vi "art联动采集V4.5.vi"() -> ()   [LabVIEW 2016]
uses:
  <vilib>/Instr/_visa.llb/VISA Configure Serial Port (Instr).vi
  <vilib>/Utility/file.llb/Write Delimited Spreadsheet (DBL).vi
panel:
  in  "hDevice 2":i32
  in  "逐行扫描":bool
  in  "定位模式":bool
  in  "X终点":dbl
  in  "Y终点":dbl
  in  "高级设置":bool
  in  "Y轴回零速度":dbl=15000.0
  in  "X轴回零速度":dbl=15000.0
  in  "细分设置":dbl=8.0
  in  "等待时间":u32=40
  in  "文件保存":path=path "C:/Users/H301/Desktop/art采集实验数据" caption="保存路径"
  out "行用时（s）":dbl
  out "time（行）":u32
  out "error out":errorcluster caption="错误输出"
  in  "退出扫描(Esc)":bool
  in  "N_Length":i32=16384
  out "M_Length":i32
  out "hDevice":i32=241832032
  out "pulDDR2Length":u32=256
  out "总用时（s）":dbl
  out "毫秒计时值":u32=3586537
  out "数组":dbl[][](array[numeric])=[[58819.77200735986, 88200.32943600747]]
  out "强度图":dbl[][](graph)=[[58819.77200735986, 88200.32943600747]]
  out "judge":dbl
  out "Xloop":dbl
  out "幅频谱":dbl[](graph)
  out "时域谱":dbl[](graph)
  out "错误输出":errorcluster
  in  "启动":bool
  in  "逐点扫描":bool
  in  "X归零":bool
  in  "Y归零":bool
  in  "Y起点":dbl
  in  "Y轴速度":dbl=9000.0
  in  "X轴速度":dbl=9000.0
  out "电机状态":bool
  in  "电机端口":refnum<visa-resource-name>="COM6"
  out "Yloop":dbl=1.0
  out "X扫描范围":dbl=150.0
  out "Y扫描范围":dbl=75.0
  out "Y序":i32
  in  "X起点":dbl
  out "Y(mm)":dbl
  out "x+y 2":dbl=3.0
  in  "Y:":dbl=1.0
  in  "精度":dbl=0.001
  in  "电机急停":bool
  out "X（mm）":dbl
  out "x+y":dbl=1.0
  in  "X:":dbl=1.0
  # "实时坐标"
  # "时域谱"
  # "频域谱"
  # "归零"
  # "扫描区域"
  # "扫描步进(mm)"
  # "X:"
  # "~"
  # "Y:"
  # "~"
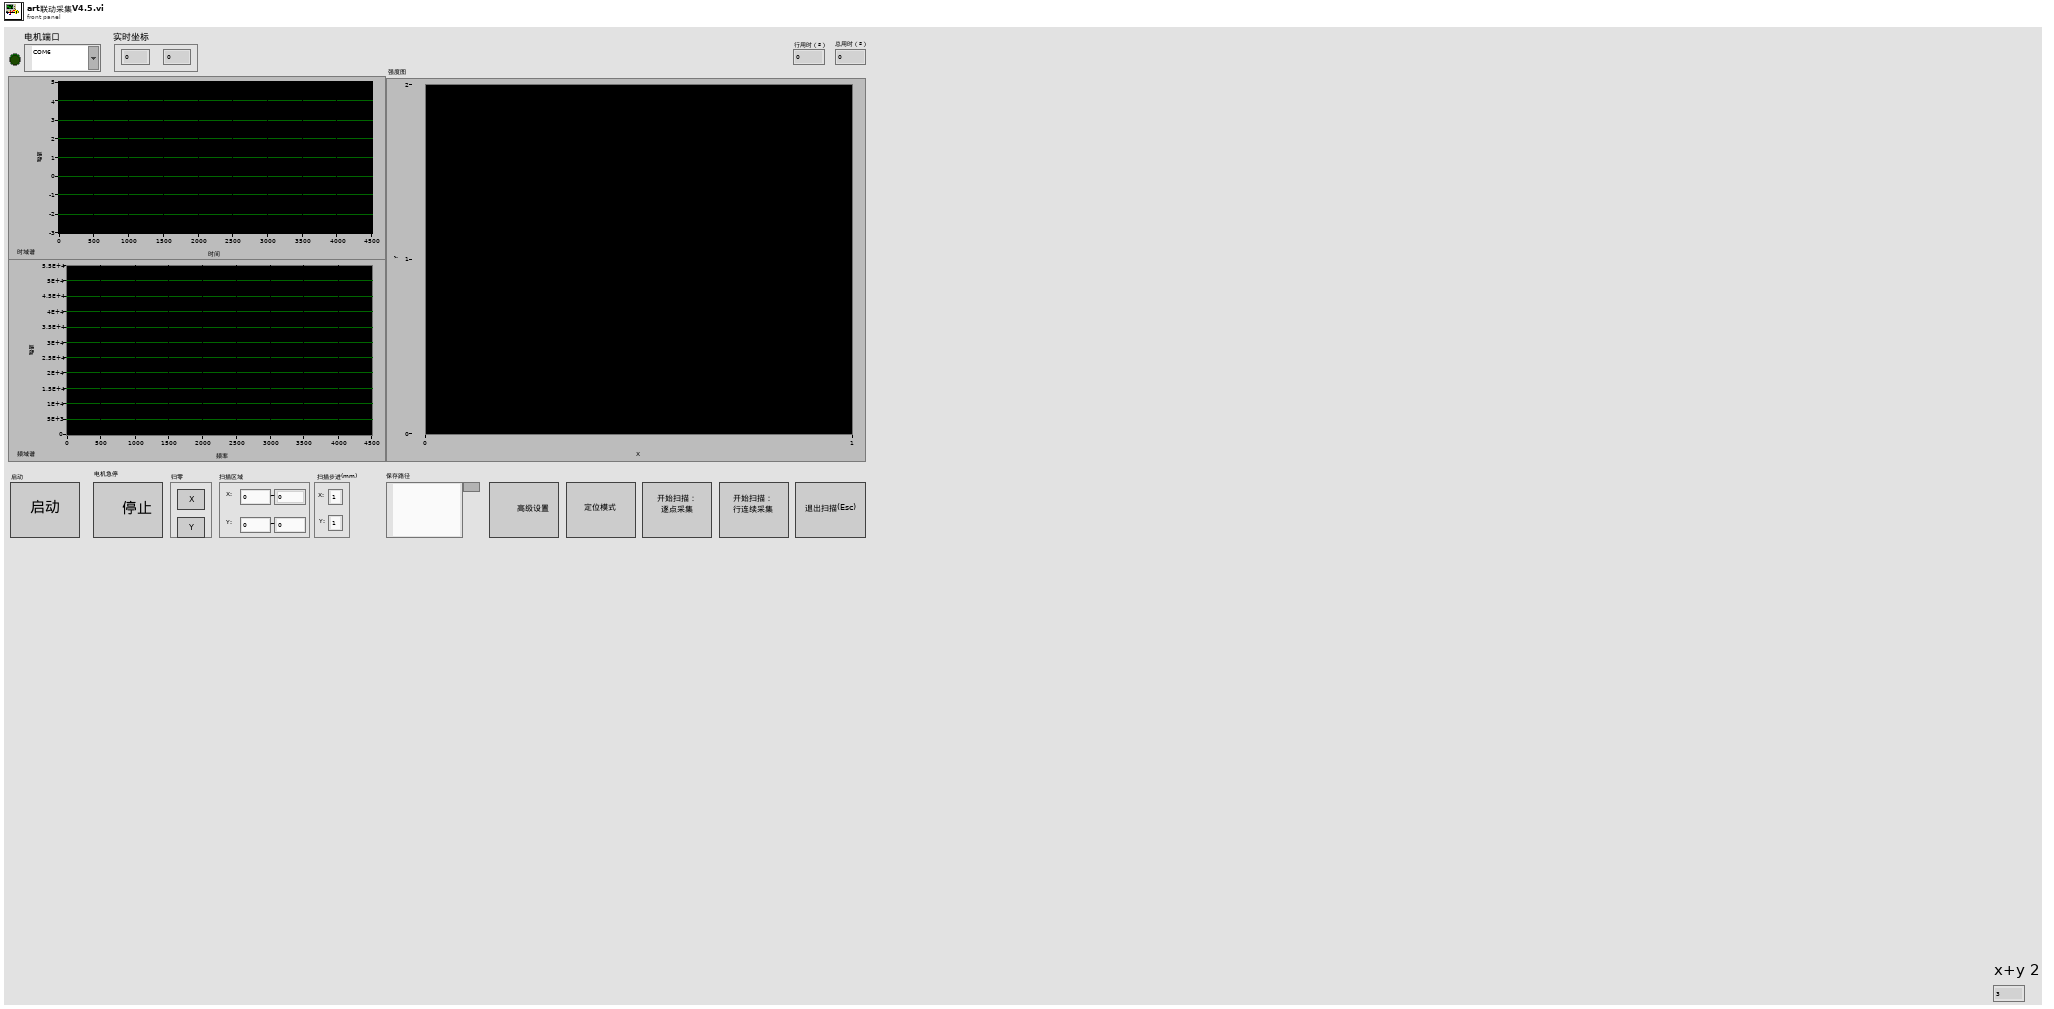
[diagram p1: front panel]
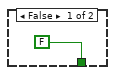
[diagram p2: hidden frame]
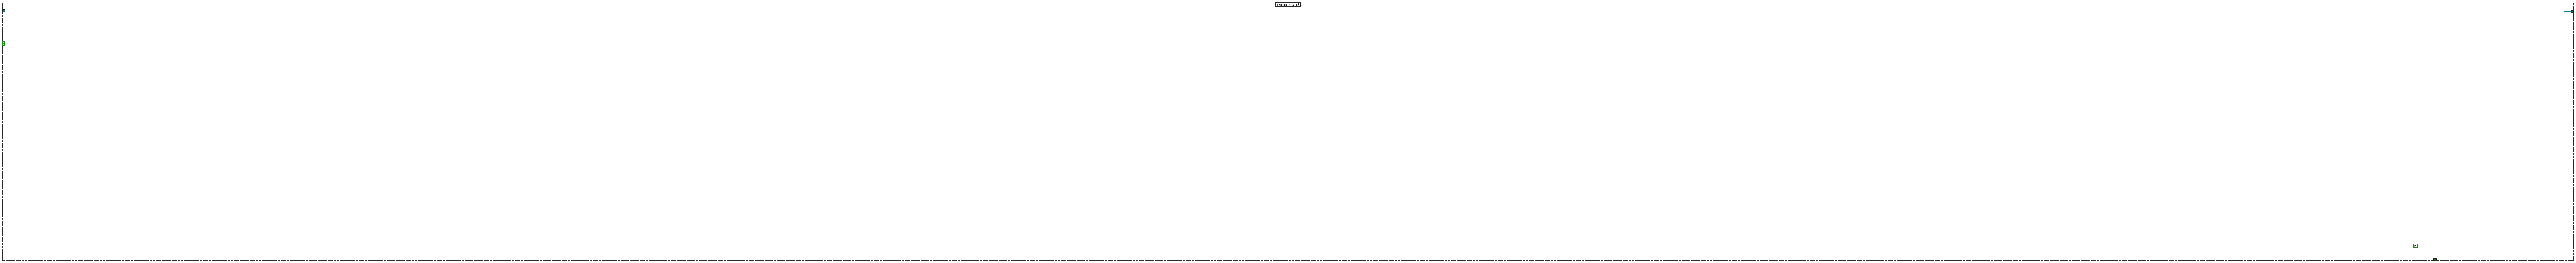
[diagram p3: hidden frame]
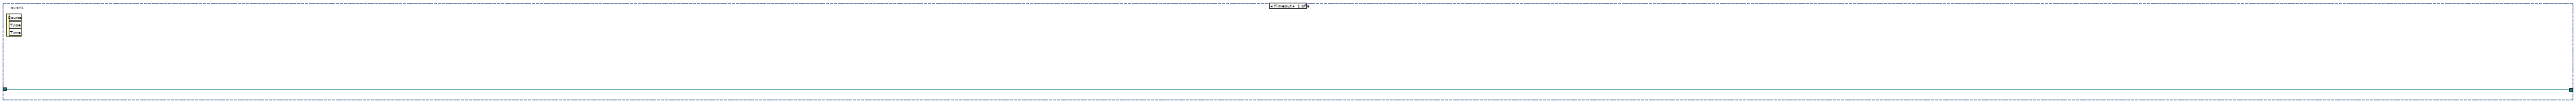
[diagram p4: hidden frame]
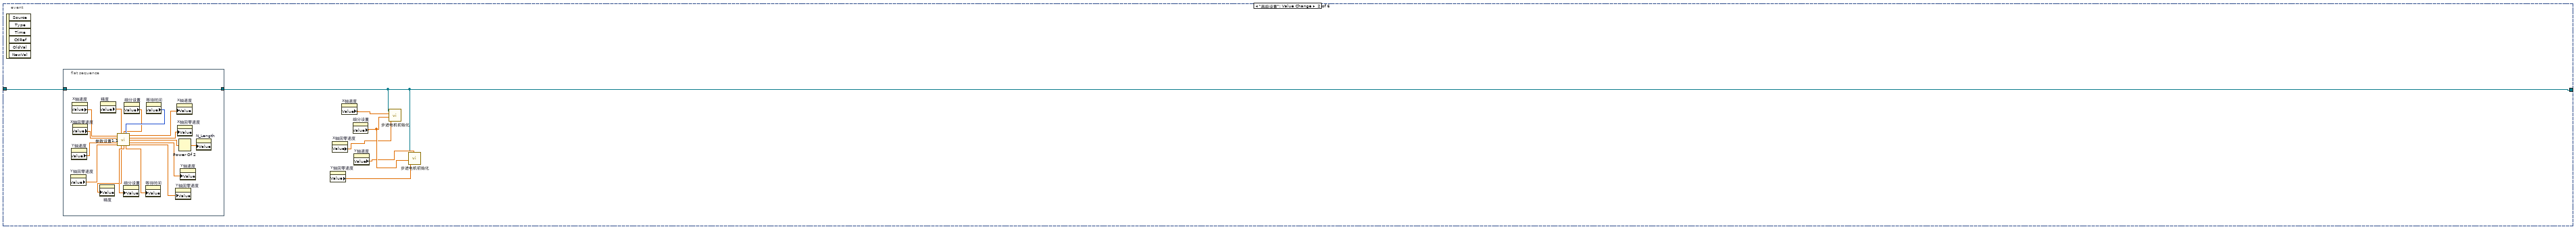
[diagram p5: hidden frame]
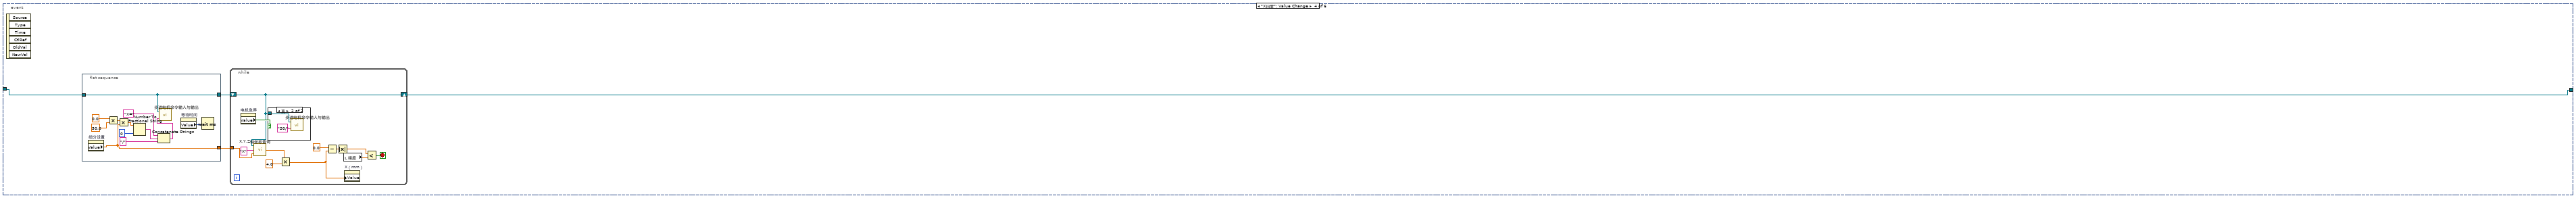
[diagram p6: hidden frame]
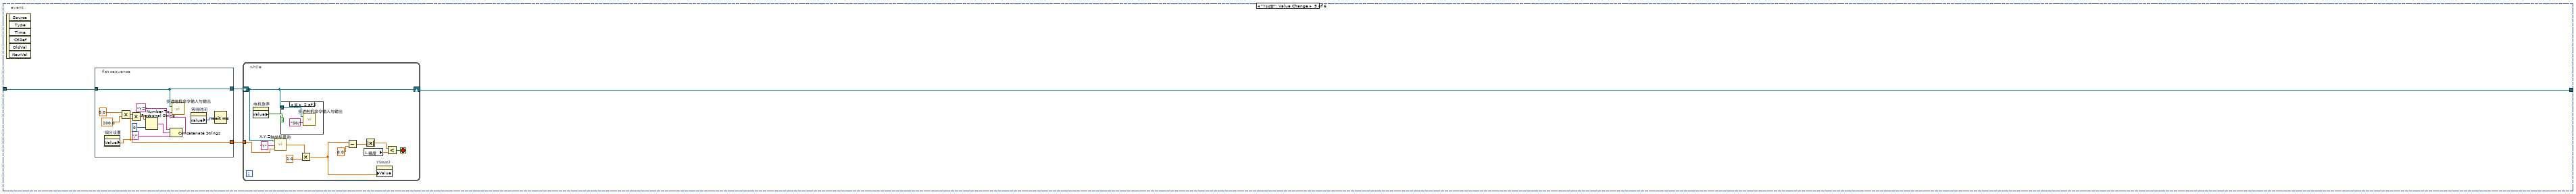
[diagram p8: hidden frame]
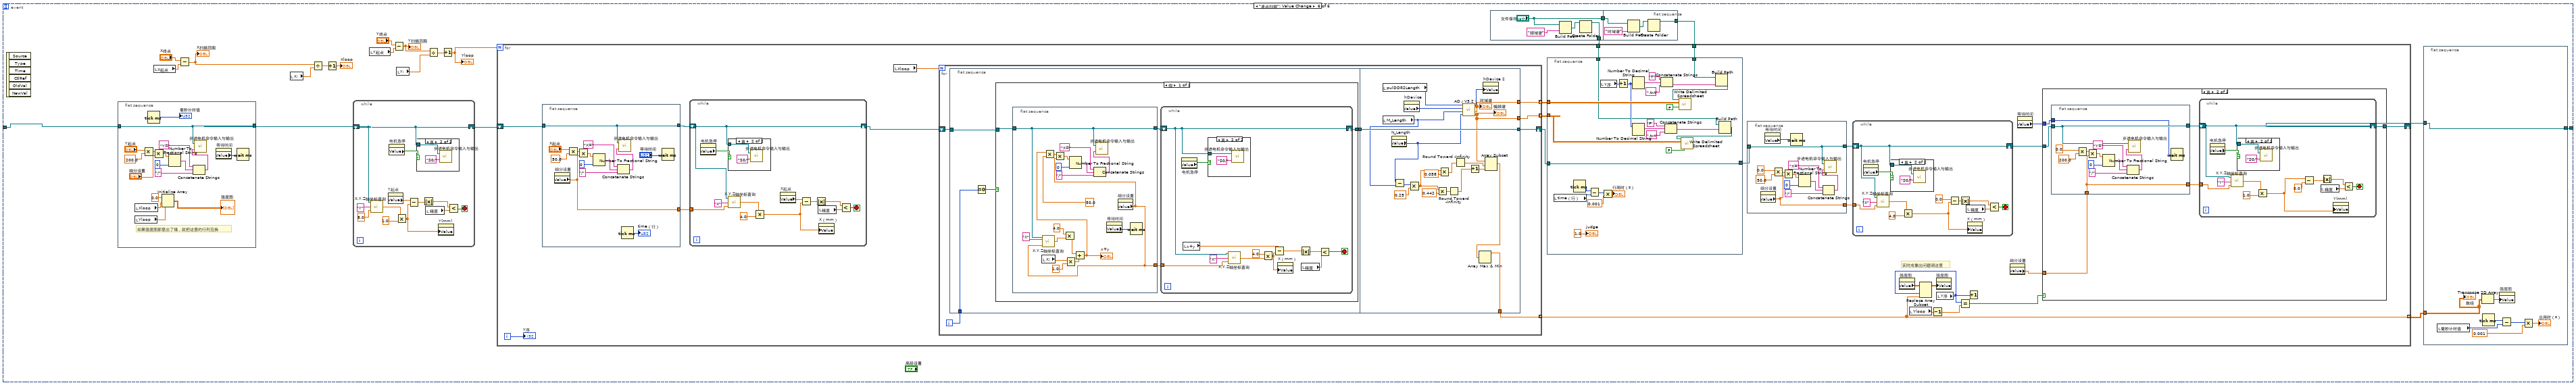
[diagram p10: hidden frame]
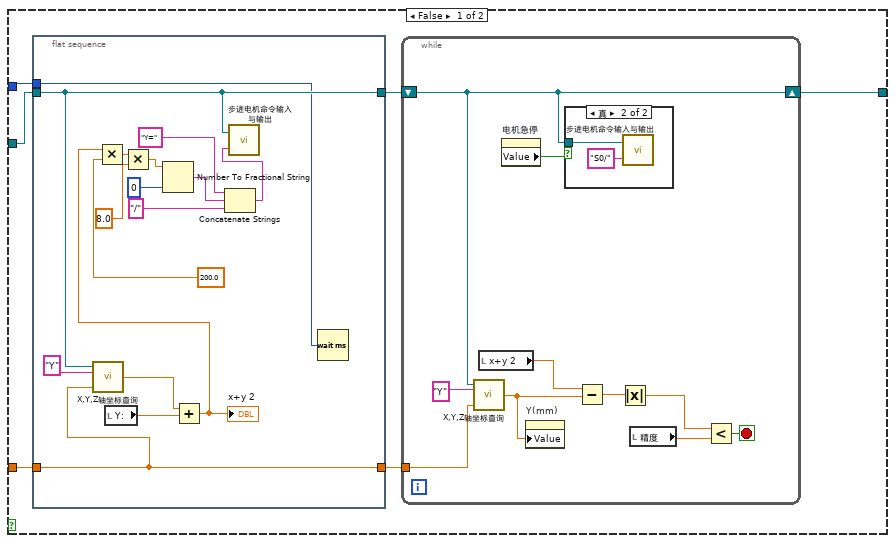
[diagram p14: hidden frame]
diagram:
  n1 = while {
    stop <- w3 stop-if-true
    n2 = case shown="真" "启动" {
      tunnel: [FALSE ("ESC") w12] -> w3
      frame False {
      }
      frame True {
        w25 = 0  # OutClockSource
        w26 = 0  # bClockSourceDir
        w28 = 10000000  # Frequency
        w29 = 0  # ClockSource
        w30 = 0  # TrigLevelVolt
        w18 = 1
        w31 = 0  # TriggerDir
        w32 = 0  # TriggerSource
        w33 = 0  # ATRTriggerChannel
        w34 = 0  # TriggerMode
        w19 = 0  # M_Length
        w35 = 1  # CouplingType
        w36 = 0  # DeviceLgcID
        w46 = u16 0 items=["无", "XON/XOFF", "RTS/CTS", "XON/XOFF & RTS/CTS", "DTR/DSR", "XON/XOFF & DTR/DSR"] ("flow control (0:none)")
        w47 = u16 10 items=["1.0"=10, "1.5"=15, "2.0"=20] ("stop bits (10: 1 bit)")
        # "3"
        # "2"
        # "1"
        n3 = call-poly "VISA Configure Serial Port"("VISA resource name"="电机端口", "baud rate (9600)"=u32 9600, "data bits (8)"=u16 8, "parity (0:none)"=enum16{"None", "Odd", "Even", "Mark", "Space"}."None", "stop bits (10: 1 bit)"=w47, "flow control (0:none)"=w46) -> ("VISA resource name out"=w38:refnum<visa-resource-name>, "error out"=→"error out":errorcluster)  [unwired: 1 in, 7 out]
        n4 = Build Array "InputRange"(w18, w18, w18, w18) -> (w17:i32[])
        n5 = dll-call lib="PTH2aabs CUsersH301Desktopart闭环扫描程序采集卡控制INFamd64PCI8502_32.dll" fn="PCI8502_CreateDevice" label="CreateDevice"("DeviceLgcID"=w36) -> (w23:i32)  [unwired: 4 in, 2 out]
        n6 = property on="细分设置" class="DigNum (严格)"() -> ("Value"=w11:dbl)  [unwired: 2 in, 2 out]
        n7 = Build Array (concatenate) "InitDeviceAD"(w28, w17, w35, w19, "N_Length", w34, w33, w32, w31, w30, w29, w26, w25) -> (w27:i32[])
        n8 = call "步进电机初始化.vi"("回零速度"="X轴回零速度", "细分设置"=w11, "X轴速度"="X轴速度", "串口通信端口"=w38) -> ()  [unwired: 2 in, 1 out]
        n9 = dll-call lib="PTH2aabs CUsersH301Desktopart闭环扫描程序采集卡控制INFamd64PCI8502_32.dll" fn="PCI8502_GetDDR2Length" label="GetDDR2Length"("hDevice"=w23, "pulDDR2Length"=u32 0) -> ("hDevice"=w22:i32, "pulDDR2Length"=→"pulDDR2Length":u32)  [unwired: 4 in, 2 out]
        n10 = call "步进电机初始化.vi"("Y轴速度"="Y轴速度", "回零速度"="Y轴回零速度", "细分设置"=w11, "串口通信端口"=w38) -> ()  [unwired: 2 in, 1 out]
        n11 = call "步进电机命令输入与输出.vi"("输入字符串"="?R/", "串口通信端口"=w38) -> ("返回字符串"=w43:string)
        n12 = dll-call lib="PTH2aabs CUsersH301Desktopart闭环扫描程序采集卡控制INFamd64PCI8502_32.dll" fn="PCI8502_InitDeviceAD" label="InitDeviceAD"("hDevice"=w22, "pADPara"=w27) -> ("hDevice"=→"hDevice":i32)  [unwired: 5 in, 2 out]
        n13 = String Subset(string=w43, offset (0)=0 ("偏移量(0)"), length (rest)=2 ("长度（剩余）")) -> (substring=w40:string)
        n14 = Equal?(x=w40, y="OK") -> (x = y?=w37:bool)
        "电机状态" <- w37
        n15 = case shown="真" w37 {
          tunnel: w38 -> [w53 w56]
          tunnel: [w53 w54] -> w13
          tunnel: [FALSE ("ESC") w55] -> w12
          frame False {
          }
          frame True {
            n16 = while {
              tunnel: ["退出扫描(Esc)"] -> w55
              shift-right: [w57] -> w54
              shift-left: w56 -> [w62]
              stop <- "退出扫描(Esc)" stop-if-true
              n17 = property on="高级设置" class="Bool"("Visible"=TRUE ("可见")) -> ()  [unwired: 2 in, 2 out]
              n18 = property on="定位模式" class="Bool"("Visible"=TRUE ("可见")) -> ()  [unwired: 2 in, 2 out]
              n19 = event shown="[2] \"定位模式\": 值改变" {
                selector: _ -> [_ _ _ _ _ _]
                dyn-events: _ -> [_ _ _ _ _ _]
                timeout: 1 -> [_ _ _ _ _ _]
                tunnel: w62 -> [w63 w70 w96 w100 w130 w177]
                tunnel: [w63 w64 w95 w98 w128 w171] -> w57
                event Timeout {
                  n20 = event-data() -> ()  [unwired: 1 in, 3 out]
                }
                event "高级设置": Value Change {
                  n21 = event-data() -> ()  [unwired: 1 in, 6 out]
                  n22 = flat-sequence {
                    tunnel: w70 -> [w73]
                    tunnel: [w73] -> w64
                    frame #0 {
                      n23 = property on="Y轴回零速度" class="DigNum (严格)"() -> ("Value"=w77:dbl)  [unwired: 2 in, 2 out]
                      n24 = property on="Y轴速度" class="DigNum (严格)"() -> ("Value"=w76:dbl)  [unwired: 2 in, 2 out]
                      n25 = property on="X轴速度" class="DigNum (严格)"() -> ("Value"=w74:dbl)  [unwired: 2 in, 2 out]
                      n26 = property on="X轴回零速度" class="DigNum (严格)"() -> ("Value"=w75:dbl)  [unwired: 2 in, 2 out]
                      n27 = property on="精度" class="DigNum (严格)"() -> ("Value"=w81:dbl)  [unwired: 2 in, 2 out]
                      n28 = property on="细分设置" class="DigNum (严格)"() -> ("Value"=w82:dbl)  [unwired: 2 in, 2 out]
                      n29 = property on="等待时间" class="DigNum (严格)"() -> ("Value"=w83:u32)  [unwired: 2 in, 2 out]
                      n30 = call "参数设置1.1.vi"("X轴速度"=w74, "精度"=w81, "细分设置"=w82, "等待时间"=w83, "X轴回零速度"=w75, "Y轴速度"=w76, "Y轴回零速度"=w77) -> ("X轴速度"=w84:dbl, "X轴回零速度"=w85:dbl, "采样阶"=w71:dbl, "Y轴速度"=w86:dbl, "精度"=w78:dbl, "细分设置"=w79:dbl, "等待时间"=w80:dbl, "Y轴回零速度"=w87:dbl)  [unwired: 1 in]
                      n31 = property on="精度" class="DigNum (严格)"("Value"=w78) -> ()  [unwired: 2 in, 2 out]
                      n32 = property on="细分设置" class="DigNum (严格)"("Value"=w79) -> ()  [unwired: 2 in, 2 out]
                      n33 = property on="等待时间" class="DigNum (严格)"("Value"=w80) -> ()  [unwired: 2 in, 2 out]
                      n34 = property on="Y轴回零速度" class="DigNum (严格)"("Value"=w87) -> ()  [unwired: 2 in, 2 out]
                      n35 = property on="X轴速度" class="DigNum (严格)"("Value"=w84) -> ()  [unwired: 2 in, 2 out]
                      n36 = property on="X轴回零速度" class="DigNum (严格)"("Value"=w85) -> ()  [unwired: 2 in, 2 out]
                      n37 = Power Of 2(x=w71) -> (2^x=w72:dbl)
                      n38 = property on="Y轴速度" class="DigNum (严格)"("Value"=w86) -> ()  [unwired: 2 in, 2 out]
                      n39 = property on="N_Length" class="DigNum (严格)"("Value"=w72) -> ()  [unwired: 2 in, 2 out]
                    }
                  }
                  n40 = property on="Y轴回零速度" class="DigNum (严格)"() -> ("Value"=w66:dbl)  [unwired: 2 in, 2 out]
                  n41 = property on="X轴回零速度" class="DigNum (严格)"() -> ("Value"=w67:dbl)  [unwired: 2 in, 2 out]
                  n42 = property on="X轴速度" class="DigNum (严格)"() -> ("Value"=w68:dbl)  [unwired: 2 in, 2 out]
                  n43 = property on="细分设置" class="DigNum (严格)"() -> ("Value"=w69:dbl)  [unwired: 2 in, 2 out]
                  n44 = property on="Y轴速度" class="DigNum (严格)"() -> ("Value"=w65:dbl)  [unwired: 2 in, 2 out]
                  n45 = call "步进电机初始化.vi"("回零速度"=w67, "细分设置"=w69, "X轴速度"=w68, "串口通信端口"=w64) -> ()  [unwired: 2 in, 1 out]
                  n46 = call "步进电机初始化.vi"("Y轴速度"=w65, "回零速度"=w66, "细分设置"=w69, "串口通信端口"=w64) -> ()  [unwired: 2 in, 1 out]
                }
                event "定位模式": Value Change {
                  n47 = event-data() -> ()  [unwired: 1 in, 6 out]
                  n48 = local read "pulDDR2Length"() -> (w92:u32)
                  n49 = local read "M_Length"() -> (w90:i32)
                  n50 = property on="hDevice" class="DigNum (严格)"() -> ("Value"=w91:i32)  [unwired: 2 in, 2 out]
                  n51 = property on="N_Length" class="DigNum (严格)"() -> ("Value"=w89:i32)  [unwired: 2 in, 2 out]
                  n52 = call "电机定位1.1.vi"("VISA I"=w96, "pulDDR2Length"=w92, "hDevice"=w91, "M-length"=w90, "N-length"=w89) -> ("hDevice out"=w88:i32, "VISA O"=w95:refnum<visa-resource-name>, "X"=w94:dbl, "Y"=w93:dbl)  [unwired: 11 in]
                  n53 = property on="hDevice 2" class="DigNum (严格)"("Value"=w88) -> ()  [unwired: 2 in, 2 out]
                  n54 = property on="X（mm）" class="DigNum (严格)"("Value"=w94) -> ()  [unwired: 2 in, 2 out]
                  n55 = property on="Y(mm)" class="DigNum (严格)"("Value"=w93) -> ()  [unwired: 2 in, 2 out]
                }
                event "X归零": Value Change {
                  n56 = event-data() -> ()  [unwired: 1 in, 6 out]
                  n57 = flat-sequence {
                    tunnel: w100 -> [w104]
                    tunnel: [w104] -> w99
                    tunnel: [w101] -> w97
                    frame #0 {
                      n58 = property on="细分设置" class="DigNum (严格)"() -> ("Value"=w101:dbl)  [unwired: 2 in, 2 out]
                      n59 = Multiply(x=0.0, y=50.0) -> (x*y=w107:dbl)
                      n60 = Multiply(x=w107, y=w101) -> (x*y=w112:dbl)
                      n61 = Number To Fractional String(number=w112, precision (6)=i16 0 ("精度(6)")) -> (F-format string=w110:string)  [unwired: 2 out]
                      n62 = Concatenate Strings("X=" ("字符串"), w110, "/" ("字符串")) -> (w105:string)
                      n63 = call "步进电机命令输入与输出.vi"("输入字符串"=w105, "串口通信端口"=w104) -> ()  [unwired: 1 out]
                      n64 = property on="等待时间" class="DigNum (严格)"() -> ("Value"=w102:u32)  [unwired: 2 in, 2 out]
                      n65 = Wait (ms)(milliseconds to wait=w102) -> ()  [unwired: 1 out]
                    }
                  }
                  n66 = while {
                    tunnel: w97 -> [w113]
                    shift-right: [w114] -> w98
                    shift-left: w99 -> [w114]
                    stop <- w120 stop-if-true
                    n67 = property on="电机急停" class="Bool (严格)"() -> ("Value"=w121:bool)  [unwired: 2 in, 2 out]
                    n68 = call "X,Y,Z轴坐标查询.vi"("细分设置"=w113, "查询坐标轴"="X", "串口通信端口"=w114) -> ("坐标(mm)"=w122:dbl)
                    n69 = case shown="真" w121 {
                      tunnel: w114 -> [_ w125]
                      frame False {
                      }
                      frame True {
                        n70 = call "步进电机命令输入与输出.vi"("输入字符串"="S0/", "串口通信端口"=w125) -> ()  [unwired: 1 out]
                      }
                    }
                    n71 = Multiply(x=w122, y=4.0 ("x")) -> (x*y=w118:dbl)
                    n72 = Subtract(x=0.0, y=w118) -> (x-y=w117:dbl)
                    n73 = Absolute Value(x=w117) -> (abs(x)=w116:dbl)
                    n74 = local read "精度"() -> (w119:dbl)
                    n75 = property on="X（mm）" class="DigNum (严格)"("Value"=w118) -> ()  [unwired: 2 in, 2 out]
                    n76 = Less?(x=w116, y=w119) -> (x < y?=w120:bool)
                  }
                }
                event "Y归零": Value Change {
                  n77 = event-data() -> ()  [unwired: 1 in, 6 out]
                  n78 = flat-sequence {
                    tunnel: w130 -> [w134]
                    tunnel: [w134] -> w129
                    tunnel: [w131] -> w127
                    frame #0 {
                      n79 = property on="细分设置" class="DigNum (严格)"() -> ("Value"=w131:dbl)  [unwired: 2 in, 2 out]
                      n80 = Multiply(x=0.0, y=200.0) -> (x*y=w137:dbl)
                      n81 = Multiply(x=w137, y=w131) -> (x*y=w142:dbl)
                      n82 = Number To Fractional String(number=w142, precision (6)=i16 0 ("精度(6)")) -> (F-format string=w140:string)  [unwired: 2 out]
                      n83 = Concatenate Strings("Y=" ("字符串"), w140, "/" ("字符串")) -> (w135:string)
                      n84 = call "步进电机命令输入与输出.vi"("输入字符串"=w135, "串口通信端口"=w134) -> ()  [unwired: 1 out]
                      n85 = property on="等待时间" class="DigNum (严格)"() -> ("Value"=w132:u32)  [unwired: 2 in, 2 out]
                      n86 = Wait (ms)(milliseconds to wait=w132) -> ()  [unwired: 1 out]
                    }
                  }
                  n87 = while {
                    tunnel: w127 -> [w143]
                    shift-right: [w144] -> w128
                    shift-left: w129 -> [w144]
                    stop <- w150 stop-if-true
                    n88 = property on="电机急停" class="Bool (严格)"() -> ("Value"=w151:bool)  [unwired: 2 in, 2 out]
                    n89 = call "X,Y,Z轴坐标查询.vi"("细分设置"=w143, "查询坐标轴"="Y", "串口通信端口"=w144) -> ("坐标(mm)"=w152:dbl)
                    n90 = case shown="真" w151 {
                      tunnel: w144 -> [_ w155]
                      frame False {
                      }
                      frame True {
                        n91 = call "步进电机命令输入与输出.vi"("输入字符串"="S0/", "串口通信端口"=w155) -> ()  [unwired: 1 out]
                      }
                    }
                    n92 = Multiply(x=w152, y=1.0 ("x")) -> (x*y=w148:dbl)
                    n93 = Subtract(x=w148, y=0.0 ("x")) -> (x-y=w146:dbl)
                    n94 = local read "精度"() -> (w149:dbl)
                    n95 = Absolute Value(x=w146) -> (abs(x)=w145:dbl)
                    n96 = property on="Y(mm)" class="DigNum (严格)"("Value"=w148) -> ()  [unwired: 2 in, 2 out]
                    n97 = Less?(x=w145, y=w149) -> (x < y?=w150:bool)
                  }
                }
                event "逐点扫描": Value Change {
                  n98 = event-data() -> ()  [unwired: 1 in, 6 out]
                  n99 = flat-sequence {
                    tunnel: w177 -> [w202]
                    tunnel: [w202] -> w167
                    frame #0 {
                      # "如果强度图那里出了错，就把这里的行列互换"
                      n100 = local read "Xloop"() -> (w197:dbl)
                      n101 = local read "Yloop"() -> (w196:dbl)
                      n102 = Multiply(x="Y起点", y=200.0) -> (x*y=w205:dbl)
                      n103 = Tick Count (ms)() -> (millisecond timer value=→"毫秒计时值":u32)
                      n104 = Multiply(x=w205, y="细分设置") -> (x*y=w210:dbl)
                      n105 = Initialize Array(0.0 ("元素"), w197, w196) -> (→"强度图":dbl[][])
                      n106 = Number To Fractional String(number=w210, precision (6)=i16 0 ("精度(6)")) -> (F-format string=w208:string)  [unwired: 2 out]
                      n107 = Concatenate Strings("Y=" ("字符串"), w208, "/" ("字符串")) -> (w203:string)
                      n108 = call "步进电机命令输入与输出.vi"("输入字符串"=w203, "串口通信端口"=w202) -> ()  [unwired: 1 out]
                      n109 = property on="等待时间" class="DigNum (严格)"() -> ("Value"=w194:u32)  [unwired: 2 in, 2 out]
                      n110 = Wait (ms)(milliseconds to wait=w194) -> ()  [unwired: 1 out]
                    }
                  }
                  n111 = local read "X起点"() -> (w163:dbl)
                  n112 = Subtract(x="X终点", y=w163) -> (x-y=w162:dbl)
                  "X扫描范围" <- w162
                  n113 = local read "X:"() -> (w170:dbl)
                  n114 = Divide(x=w162, y=w170) -> (x/y=w168:dbl)
                  n115 = Increment(x=w168) -> (x+1=→"Xloop":dbl)
                  n116 = while {
                    shift-right: [w211] -> w159
                    shift-left: w167 -> [w211]
                    stop <- w216 stop-if-true
                    n117 = call "X,Y,Z轴坐标查询.vi"("细分设置"=8.0, "查询坐标轴"="Y", "串口通信端口"=w211) -> ("坐标(mm)"=w218:dbl)
                    n118 = property on="Y起点" class="DigNum (严格)"() -> ("Value"=w220:dbl)  [unwired: 2 in, 2 out]
                    n119 = property on="电机急停" class="Bool (严格)"() -> ("Value"=w217:bool)  [unwired: 2 in, 2 out]
                    n120 = Multiply(x=w218, y=1.0 ("x")) -> (x*y=w214:dbl)
                    n121 = Subtract(x=w220, y=w214) -> (x-y=w213:dbl)
                    n122 = case shown="真" w217 {
                      tunnel: w211 -> [_ w223]
                      frame False {
                      }
                      frame True {
                        n123 = call "步进电机命令输入与输出.vi"("输入字符串"="S0/", "串口通信端口"=w223) -> ()  [unwired: 1 out]
                      }
                    }
                    n124 = Absolute Value(x=w213) -> (abs(x)=w212:dbl)
                    n125 = local read "精度"() -> (w215:dbl)
                    n126 = property on="Y(mm)" class="DigNum (严格)"("Value"=w214) -> ()  [unwired: 2 in, 2 out]
                    n127 = Less?(x=w212, y=w215) -> (x < y?=w216:bool)
                  }
                  n128 = local read "Y起点"() -> (w165:dbl)
                  n129 = Subtract(x="Y终点", y=w165) -> (x-y=w161:dbl)
                  "Y扫描范围" <- w161
                  n130 = local read "Y:"() -> (w176:dbl)
                  n131 = Divide(x=w161, y=w176) -> (x/y=w175:dbl)
                  n132 = Increment(x=w175) -> (x+1=w174:dbl)
                  "Yloop" <- w174
                  n133 = for {
                    N: w174 -> [_]
                    shift-right: [w247] -> w173
                    shift-left: w159 -> [w227]
                    tunnel: [w229] -> w172 mode=indexing
                    tunnel: w157 -> [w233]
                    tunnel: w160 -> [w232]
                    i -> [w248]
                    # "实时成像出问题调这里"
                    n134 = flat-sequence {
                      tunnel: w227 -> [w305]
                      tunnel: [w305] -> w246
                      tunnel: [w301] -> w237
                      frame #0 {
                        n135 = property on="细分设置" class="DigNum (严格)"() -> ("Value"=w301:dbl)  [unwired: 2 in, 2 out]
                        n136 = Multiply(x="X起点", y=50.0) -> (x*y=w308:dbl)
                        n137 = Multiply(x=w308, y=w301) -> (x*y=w313:dbl)
                        n138 = Number To Fractional String(number=w313, precision (6)=i16 0 ("精度(6)")) -> (F-format string=w311:string)  [unwired: 2 out]
                        n139 = Concatenate Strings("X=" ("字符串"), w311, "/" ("字符串")) -> (w306:string)
                        n140 = call "步进电机命令输入与输出.vi"("输入字符串"=w306, "串口通信端口"=w305) -> ()  [unwired: 1 out]
                        n141 = Tick Count (ms)() -> (millisecond timer value=→"time（行）":u32)
                        n142 = Wait (ms)(milliseconds to wait="等待时间") -> ()  [unwired: 1 out]
                      }
                    }
                    n143 = while {
                      tunnel: w237 -> [w315]
                      shift-right: [w314] -> w225
                      shift-left: w246 -> [w314]
                      stop <- w320 stop-if-true
                      n144 = property on="电机急停" class="Bool (严格)"() -> ("Value"=w321:bool)  [unwired: 2 in, 2 out]
                      n145 = case shown="真" w321 {
                        tunnel: w314 -> [_ w326]
                        frame False {
                        }
                        frame True {
                          n146 = call "步进电机命令输入与输出.vi"("输入字符串"="S0/", "串口通信端口"=w326) -> ()  [unwired: 1 out]
                        }
                      }
                      n147 = call "X,Y,Z轴坐标查询.vi"("细分设置"=w315, "查询坐标轴"="X", "串口通信端口"=w314) -> ("坐标(mm)"=w322:dbl)
                      n148 = Multiply(x=w322, y=4.0 ("x")) -> (x*y=w318:dbl)
                      n149 = property on="X起点" class="DigNum (严格)"() -> ("Value"=w324:dbl)  [unwired: 2 in, 2 out]
                      n150 = Subtract(x=w324, y=w318) -> (x-y=w317:dbl)
                      n151 = Absolute Value(x=w317) -> (abs(x)=w316:dbl)
                      n152 = local read "精度"() -> (w319:dbl)
                      n153 = property on="X（mm）" class="DigNum (严格)"("Value"=w318) -> ()  [unwired: 2 in, 2 out]
                      n154 = Less?(x=w316, y=w319) -> (x < y?=w320:bool)
                    }
                    n155 = local read "Xloop"() -> (w238:dbl)
                    n156 = for {
                      N: w238 -> [_]
                      shift-right: [w399] -> w226
                      shift-left: w225 -> [w394]
                      tunnel: [w398] -> w245 mode=indexing
                      tunnel: [w397] -> w244 mode=indexing
                      tunnel: [w396] -> w229 mode=indexing
                      i -> [w395]
                      n157 = flat-sequence {
                        tunnel: w394 -> [w404]
                        tunnel: [w403] -> w400
                        tunnel: w395 -> [w401]
                        tunnel: [w462] -> w399
                        tunnel: w400 -> [w462]
                        tunnel: [w461] -> w398
                        tunnel: [w460] -> w397
                        tunnel: [w458] -> w396
                        frame #0 {
                          n158 = Equal To 0?(x=w401) -> (x = 0?=w402:bool)
                          n159 = case shown="假" w402 {
                            tunnel: w404 -> [w407 w442]
                            tunnel: [w406 w442] -> w403
                            frame False {
                              n160 = flat-sequence {
                                tunnel: w407 -> [w417]
                                tunnel: [w417] -> w408
                                tunnel: [w409] -> w405
                                frame #0 {
                                n161 = local read "X:"() -> (w411:dbl)
                                n162 = Multiply(x=w411, y=1.0 ("x")) -> (x*y=w416:dbl)
                                n163 = property on="等待时间" class="DigNum (严格)"() -> ("Value"=w410:u32)  [unwired: 2 in, 2 out]
                                n164 = property on="细分设置" class="DigNum (严格)"() -> ("Value"=w409:dbl)  [unwired: 2 in, 2 out]
                                n165 = call "X,Y,Z轴坐标查询.vi"("细分设置"=w409, "查询坐标轴"="X", "串口通信端口"=w417) -> ("坐标(mm)"=w413:dbl)
                                n166 = Multiply(x=4.0, y=w413) -> (x*y=w412:dbl)
                                n167 = Add(x=w412, y=w416) -> (x+y=w419:dbl)
                                "x+y" <- w419
                                n168 = Multiply(x=w419, y=50.0) -> (x*y=w422:dbl)
                                n169 = Multiply(x=w422, y=w409) -> (x*y=w427:dbl)
                                n170 = Number To Fractional String(number=w427, precision (6)=i16 0 ("精度(6)")) -> (F-format string=w425:string)  [unwired: 2 out]
                                n171 = Concatenate Strings("X=" ("字符串"), w425, "/" ("字符串")) -> (w420:string)
                                n172 = call "步进电机命令输入与输出.vi"("输入字符串"=w420, "串口通信端口"=w417) -> ()  [unwired: 1 out]
                                n173 = Wait (ms)(milliseconds to wait=w410) -> ()  [unwired: 1 out]
                                }
                              }
                              n174 = while {
                                tunnel: w405 -> [w428]
                                shift-right: [w437] -> w406
                                shift-left: w408 -> [w437]
                                stop <- w436 stop-if-true
                                n175 = property on="电机急停" class="Bool (严格)"() -> ("Value"=w434:bool)  [unwired: 2 in, 2 out]
                                n176 = local read "x+y"() -> (w438:dbl)
                                n177 = case shown="真" w434 {
                                tunnel: w437 -> [_ w440]
                                frame False {
                                }
                                frame True {
                                n178 = call "步进电机命令输入与输出.vi"("输入字符串"="S0/", "串口通信端口"=w440) -> ()  [unwired: 1 out]
                                }
                                }
                                n179 = call "X,Y,Z轴坐标查询.vi"("细分设置"=w428, "查询坐标轴"="X", "串口通信端口"=w437) -> ("坐标(mm)"=w432:dbl)
                                n180 = Multiply(x=4.0, y=w432) -> (x*y=w431:dbl)
                                n181 = Subtract(x=w438, y=w431) -> (x-y=w430:dbl)
                                n182 = property on="X（mm）" class="DigNum (严格)"("Value"=w431) -> ()  [unwired: 2 in, 2 out]
                                n183 = Absolute Value(x=w430) -> (abs(x)=w429:dbl)
                                n184 = local read "精度"() -> (w433:dbl)
                                n185 = Less?(x=w429, y=w433) -> (x < y?=w436:bool)
                              }
                            }
                            frame True {
                            }
                          }
                        }
                        frame #1 {
                          n186 = local read "pulDDR2Length"() -> (w457:u32)
                          n187 = local read "M_Length"() -> (w456:i32)
                          n188 = property on="N_Length" class="DigNum (严格)"() -> ("Value"=w445:i32)  [unwired: 2 in, 2 out]
                          n189 = Subtract(x=w445, y=w456) -> (x-y=w454:i32)
                          n190 = property on="hDevice" class="DigNum (严格)"() -> ("Value"=w443:i32)  [unwired: 2 in, 2 out]
                          n191 = Multiply(x=w454, y=0.25) -> (x*y=w447:dbl)
                          n192 = Multiply(x=w447, y=0.442) -> (x*y=w449:dbl)
                          n193 = Multiply(x=w447, y=0.058) -> (x*y=w451:dbl)
                          n194 = Round Toward -Infinity(1:w449) -> (0:w446:dbl)
                          n195 = Round Toward -Infinity(1:w451) -> (0:w450:dbl)
                          n196 = call "AD（V3.2）.vi"("N-length"=w445, "M-length"=w456, "hDevice"=w443, "pulDDR2Length"=w457) -> ("幅频谱"=w460:dbl[], "时域谱"=w461:dbl[], "hDevice out"=w444:i32)  [unwired: 5 in]
                          "时域谱" <- w461
                          "幅频谱" <- w460
                          n197 = Increment(x=w446) -> (x+1=w453:dbl)
                          n198 = property on="hDevice 2" class="DigNum (严格)"("Value"=w444) -> ()  [unwired: 2 in, 2 out]
                          n199 = Array Subset(array=w460, index=w450, length=w453) -> (w459:dbl[])
                          n200 = Array Max & Min(array=w459) -> (max value=w458:dbl)  [unwired: 3 out]
                        }
                      }
                    }
                    n201 = flat-sequence {
                      tunnel: w244 -> [w282]
                      tunnel: w245 -> [w290]
                      tunnel: w226 -> [w299]
                      tunnel: [w299] -> w240
                      tunnel: w233 -> [w277]
                      tunnel: w232 -> [w276]
                      frame #0 {
                        n202 = local read "time（行）"() -> (w298:u32)
                        n203 = Tick Count (ms)() -> (millisecond timer value=w294:u32)
                        n204 = Subtract(x=w294, y=w298) -> (x-y=w297:u32)
                        n205 = local read "Y序"() -> (w278:i32)
                        n206 = Multiply(x=w297, y=0.001) -> (x*y=→"行用时（s）":dbl)
                        n207 = Increment(x=w278) -> (x+1=w279:i32)
                        n208 = Number To Decimal String(number=w279) -> (decimal integer string=w288:string)  [unwired: 1 in]
                        n209 = Number To Decimal String(number=w279) -> (decimal integer string=w287:string)  [unwired: 1 in]
                        n210 = Concatenate Strings("T" ("字符串"), w288, ".txt" ("字符串")) -> (w291:string)
                        n211 = Concatenate Strings("F" ("字符串"), w287, ".txt" ("字符串")) -> (w285:string)
                        n212 = Build Path(base path=w277, name or relative path=w291) -> (appended path=w293:path)
                        n213 = call-poly <vilib>:"Write Delimited Spreadsheet.vi"("file path (dialog if empty)"=w293, "2D data"=w290, "transpose? (no:F)"=FALSE) -> ()  [unwired: 11 in, 2 out]
                        n214 = Build Path(base path=w276, name or relative path=w285) -> (appended path=w283:path)
                        n215 = call-poly <vilib>:"Write Delimited Spreadsheet.vi"("file path (dialog if empty)"=w283, "2D data"=w282, "transpose? (no:F)"=FALSE) -> ()  [unwired: 11 in, 2 out]
                        "judge" <- 1.0
                      }
                    }
                    n216 = flat-sequence {
                      tunnel: w240 -> [w253]
                      tunnel: [w253] -> w241
                      tunnel: [w251] -> w236
                      frame #0 {
                        n217 = property on="细分设置" class="DigNum (严格)"() -> ("Value"=w251:dbl)  [unwired: 2 in, 2 out]
                        n218 = property on="等待时间" class="DigNum (严格)"() -> ("Value"=w250:u32)  [unwired: 2 in, 2 out]
                        n219 = Multiply(x=0.0, y=50.0) -> (x*y=w256:dbl)
                        n220 = Multiply(x=w256, y=w251) -> (x*y=w261:dbl)
                        n221 = Wait (ms)(milliseconds to wait=w250) -> ()  [unwired: 1 out]
                        n222 = Number To Fractional String(number=w261, precision (6)=i16 0 ("精度(6)")) -> (F-format string=w259:string)  [unwired: 2 out]
                        n223 = Concatenate Strings("X=" ("字符串"), w259, "/" ("字符串")) -> (w254:string)
                        n224 = call "步进电机命令输入与输出.vi"("输入字符串"=w254, "串口通信端口"=w253) -> ()  [unwired: 1 out]
                      }
                    }
                    n225 = while {
                      tunnel: w236 -> [w262]
                      shift-right: [w263] -> w239
                      shift-left: w241 -> [w263]
                      stop <- w269 stop-if-true
                      n226 = property on="电机急停" class="Bool (严格)"() -> ("Value"=w270:bool)  [unwired: 2 in, 2 out]
                      n227 = call "X,Y,Z轴坐标查询.vi"("细分设置"=w262, "查询坐标轴"="X", "串口通信端口"=w263) -> ("坐标(mm)"=w271:dbl)
                      n228 = case shown="真" w270 {
                        tunnel: w263 -> [_ w274]
                        frame False {
                        }
                        frame True {
                          n229 = call "步进电机命令输入与输出.vi"("输入字符串"="S0/", "串口通信端口"=w274) -> ()  [unwired: 1 out]
                        }
                      }
                      n230 = Multiply(x=w271, y=4.0 ("x")) -> (x*y=w267:dbl)
                      n231 = Subtract(x=0.0, y=w267) -> (x-y=w266:dbl)
                      n232 = Absolute Value(x=w266) -> (abs(x)=w265:dbl)
                      n233 = local read "精度"() -> (w268:dbl)
                      n234 = property on="X（mm）" class="DigNum (严格)"("Value"=w267) -> ()  [unwired: 2 in, 2 out]
                      n235 = Less?(x=w265, y=w268) -> (x < y?=w269:bool)
                    }
                    n236 = property on="强度图" class="IntGraph (严格)"() -> ("Value"=w230:dbl[][])  [unwired: 2 in, 2 out]
                    n237 = local read "Yloop"() -> (w242:dbl)
                    n238 = Decrement(x=w242) -> (x-1=w243:dbl)
                    n239 = local read "Y序"() -> (w228:i32)
                    n240 = Replace Array Subset(array=w230, new element=w229, index (col)=w228) -> (w231:dbl[][])  [unwired: 1 in]
                    n241 = property on="强度图" class="IntGraph (严格)"("Value"=w231) -> ()  [unwired: 2 in, 2 out]
                    n242 = Equal?(x=w228, y=w243) -> (x = y?=w249:bool)
                    n243 = Increment(x=w228) -> ()  [unwired: 1 out]
                    n244 = property on="细分设置" class="DigNum (严格)"() -> ("Value"=w234:dbl)  [unwired: 2 in, 2 out]
                    n245 = property on="等待时间" class="DigNum (严格)"() -> ("Value"=w235:u32)  [unwired: 2 in, 2 out]
                    n246 = case shown="真" w249 {
                      tunnel: w239 -> [w333 w365]
                      tunnel: [w331 w366] -> w247
                      tunnel: w235 -> [w329 w363]
                      tunnel: w234 -> [w328 w362]
                      frame False {
                        n247 = flat-sequence {
                          tunnel: w333 -> [w336]
                          tunnel: [w336] -> w332
                          tunnel: [w334] -> w330
                          tunnel: w329 -> [w335]
                          tunnel: w328 -> [w334]
                          frame #0 {
                            n248 = call "X,Y,Z轴坐标查询.vi"("细分设置"=w334, "查询坐标轴"="Y", "串口通信端口"=w336) -> ("坐标(mm)"=w338:dbl)
                            n249 = local read "Y:"() -> (w337:dbl)
                            n250 = Add(x=w338, y=w337) -> (x+y=w340:dbl)
                            "x+y 2" <- w340
                            n251 = Multiply(x=w340, y=200.0) -> (x*y=w344:dbl)
                            n252 = Multiply(x=w344, y=8.0 ("细分设置")) -> (x*y=w349:dbl)
                            n253 = Number To Fractional String(number=w349, precision (6)=i16 0 ("精度(6)")) -> (F-format string=w347:string)  [unwired: 2 out]
                            n254 = Concatenate Strings("Y=" ("字符串"), w347, "/" ("字符串")) -> (w342:string)
                            n255 = call "步进电机命令输入与输出.vi"("输入字符串"=w342, "串口通信端口"=w336) -> ()  [unwired: 1 out]
                            n256 = Wait (ms)(milliseconds to wait=w335) -> ()  [unwired: 1 out]
                          }
                        }
                        n257 = while {
                          tunnel: w330 -> [w350]
                          shift-right: [w351] -> w331
                          shift-left: w332 -> [w351]
                          stop <- w357 stop-if-true
                          n258 = call "X,Y,Z轴坐标查询.vi"("细分设置"=w350, "查询坐标轴"="Y", "串口通信端口"=w351) -> ("坐标(mm)"=w355:dbl)
                          n259 = local read "x+y 2"() -> (w358:dbl)
                          n260 = property on="电机急停" class="Bool (严格)"() -> ("Value"=w354:bool)  [unwired: 2 in, 2 out]
                          n261 = property on="Y(mm)" class="DigNum (严格)"("Value"=w355) -> ()  [unwired: 2 in, 2 out]
                          n262 = case shown="真" w354 {
                            tunnel: w351 -> [_ w360]
                            frame False {
                            }
                            frame True {
                              n263 = call "步进电机命令输入与输出.vi"("输入字符串"="S0/", "串口通信端口"=w360) -> ()  [unwired: 1 out]
                            }
                          }
                          n264 = Subtract(x=w358, y=w355) -> (x-y=w353:dbl)
                          n265 = Absolute Value(x=w353) -> (abs(x)=w352:dbl)
                          n266 = local read "精度"() -> (w356:dbl)
                          n267 = Less?(x=w352, y=w356) -> (x < y?=w357:bool)
                        }
                      }
                      frame True {
                        n268 = flat-sequence {
                          tunnel: [w370] -> _
                          tunnel: [w370] -> w367
                          tunnel: w365 -> [w370]
                          tunnel: [w368] -> w364
                          tunnel: w363 -> [w369]
                          tunnel: w362 -> [w368]
                          frame #0 {
                            n269 = Multiply(x=0.0, y=200.0) -> (x*y=w374:dbl)
                            n270 = Multiply(x=w374, y=w368) -> (x*y=w379:dbl)
                            n271 = Number To Fractional String(number=w379, precision (6)=i16 0 ("精度(6)")) -> (F-format string=w377:string)  [unwired: 2 out]
                            n272 = Concatenate Strings("Y=" ("字符串"), w377, "/" ("字符串")) -> (w372:string)
                            n273 = call "步进电机命令输入与输出.vi"("输入字符串"=w372, "串口通信端口"=w370) -> ()  [unwired: 1 out]
                            n274 = Wait (ms)(milliseconds to wait=w369) -> ()  [unwired: 1 out]
                          }
                        }
                        n275 = while {
                          tunnel: w364 -> [w380]
                          shift-right: [w381] -> w366
                          shift-left: w367 -> [w381]
                          stop <- w387 stop-if-true
                          n276 = property on="电机急停" class="Bool (严格)"() -> ("Value"=w388:bool)  [unwired: 2 in, 2 out]
                          n277 = call "X,Y,Z轴坐标查询.vi"("细分设置"=w380, "查询坐标轴"="Y", "串口通信端口"=w381) -> ("坐标(mm)"=w389:dbl)
                          n278 = case shown="真" w388 {
                            tunnel: w381 -> [_ w392]
                            frame False {
                            }
                            frame True {
                              n279 = call "步进电机命令输入与输出.vi"("输入字符串"="S0/", "串口通信端口"=w392) -> ()  [unwired: 1 out]
                            }
                          }
                          n280 = Multiply(x=w389, y=1.0 ("x")) -> (x*y=w385:dbl)
                          n281 = Subtract(x=w385, y=0.0 ("x")) -> (x-y=w383:dbl)
                          n282 = local read "精度"() -> (w386:dbl)
                          n283 = Absolute Value(x=w383) -> (abs(x)=w382:dbl)
                          n284 = property on="Y(mm)" class="DigNum (严格)"("Value"=w385) -> ()  [unwired: 2 in, 2 out]
                          n285 = Less?(x=w382, y=w386) -> (x < y?=w387:bool)
                        }
                      }
                    }
                    "Y序" <- w248
                  }
                  n286 = flat-sequence {
                    tunnel: [w178] -> w160
                    tunnel: ["文件保存"] -> w158
                    tunnel: w158 -> [w183]
                    tunnel: [w182] -> w157
                    frame #0 {
                      n287 = Build Path(base path="文件保存", name or relative path="频域谱" ("名称或相对路径")) -> (appended path=w181:path)
                      n288 = Create Folder(path (use dialog)=w181) -> (created path=w178:path)  [unwired: 2 in, 2 out]
                    }
                    frame #1 {
                      n289 = Build Path(base path=w183, name or relative path="时域谱" ("名称或相对路径")) -> (appended path=w184:path)
                      n290 = Create Folder(path (use dialog)=w184) -> (created path=w182:path)  [unwired: 2 in, 2 out]
                    }
                  }
                  n291 = flat-sequence {
                    tunnel: w173 -> [w188]
                    tunnel: w172 -> [w187]
                    tunnel: [w188] -> w171
                    frame #0 {
                      n292 = local read "毫秒计时值"() -> (w192:u32)
                      n293 = Transpose 2D Array(2D array=w187) -> (transposed array=w186:dbl[][])
                      n294 = Tick Count (ms)() -> (millisecond timer value=w193:u32)
                      n295 = property on="强度图" class="IntGraph (严格)"("Value"=w186) -> ()  [unwired: 2 in, 2 out]
                      n296 = Subtract(x=w193, y=w192) -> (x-y=w189:u32)
                      n297 = Multiply(x=w189, y=0.001) -> (x*y=→"总用时（s）":dbl)
                      "数组" <- w187
                    }
                  }
                }
              }
            }
          }
        }
        n298 = dll-call lib="PTH2]abs CUsersH301Desktopart闭环扫描程序采集卡控制INFamd64\nPCI8502_32" fn="PCI8502_ReleaseDeviceAD" label="ReleaseDeviceAD"("hDevice"="hDevice 2") -> ("hDevice"=w15:i32)  [unwired: 4 in, 2 out]
        n299 = VISA Close(VISA resource name=w13) -> (error out=→"错误输出":errorcluster)  [unwired: 1 in]
        n300 = dll-call lib="PTH2]abs CUsersH301Desktopart闭环扫描程序采集卡控制INFamd64\nPCI8502_32" fn="PCI8502_ReleaseDevice" label="ReleaseDevice"("hDevice"=w15) -> ()  [unwired: 5 in, 2 out]
        "M_Length" <- w19
      }
    }
  }
  n301 = property on="高级设置" class="Bool"("Visible"=FALSE ("可见")) -> ()  [unwired: 2 in, 2 out]
  n302 = property on="定位模式" class="Bool"("Visible"=FALSE ("可见")) -> ()  [unwired: 2 in, 2 out]
